vi "ElevatorFeedForward.vi"(9 "Elevator State":string) -> (2 "Feed Forward Contribution":dbl)   [LabVIEW 2018]
uses:
  Inputs_DriverStation.vi
  SensorReadings.vi
  RobotStates.vi
panel:
  in  "Stage 2 Position (in)":dbl=61.7
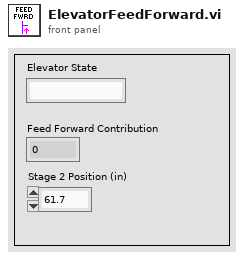
[diagram p1: front panel]
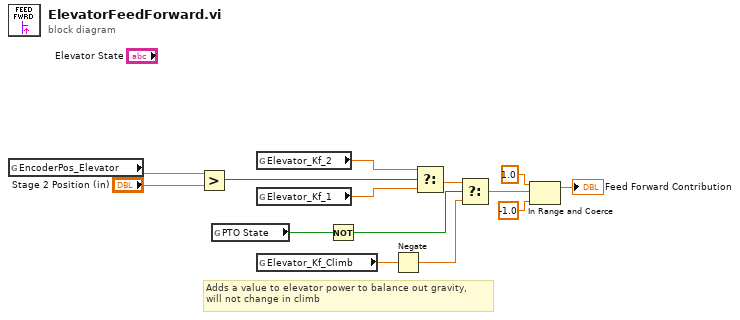
[diagram p0: block diagram]
diagram:
  # "Adds a value to elevator power to balance out gravity, \nwill not change in climb"
  n1 = global read "SensorReadings.vi" "EncoderPos_Elevator"() -> (w9:dbl)
  n2 = Greater?(x=w9, y="Stage 2 Position (in)") -> (0:w10:bool)
  n3 = global read "RobotStates.vi" "PTO State"() -> (w3:bool)
  n4 = global read "Inputs_DriverStation.vi" "Elevator_Kf_2"() -> (w4:dbl)
  n5 = global read "Inputs_DriverStation.vi" "Elevator_Kf_1"() -> (w11:dbl)
  n6 = global read "Inputs_DriverStation.vi" "Elevator_Kf_Climb"() -> (w5:dbl)
  n7 = Not(x=w3) -> (.not. x?=w2:bool)
  n8 = Negate(x=w5) -> (-x=w1:dbl)
  n9 = Select(t=w4, s=w10, f=w11) -> (s? t:f=w7:dbl)
  n10 = Select(t=w7, s=w2, f=w1) -> (s? t:f=w6:dbl)
  n11 = In Range and Coerce(upper limit=1.0, x=w6, lower limit=-1.0) -> (coerced(x)=→"Feed Forward Contribution":dbl)  [unwired: 1 out]
